vi "SENS_SWE_GEN.vi"(0 "VISA IN":refnum<visa-resource-name>, 1 "Source Frq. Mode":string(combo)="STEPped", 5 "error in":errorcluster, 7 "Channel":i32=1) -> (14 "VISA Out":refnum<visa-resource-name>, 19 "error out":errorcluster)   [LabVIEW 2018, in "PNA-X.lvlib"]
doc: "SENSe<cnum>:SWEep:GENeration <char> \n(Read-Write) Sets sweep as Stepped or Analog. \nParameters \n<cnum> Any existing channel number. If unspecified, value is set to 1 \n<char> Choose from: \nSTEPped - source frequency is CONSTANT during measurement of eah displayed \npoint. More accurate than ANALog. Dwell time can be set in this mode. \nANALog - source frequency is continuously RAMPING during measurement of each \ndisplayed point. Faster than STEPped. Sweep time (not dwell time) can be set in this \nmode. \nExamples SENS:SWE:GEN STEP \nsense2:sweep:generation analog \nQuery Syntax SENSe<cnum>:SWEep:GENeration? \nReturn Type Character"
uses:
  PNA-X.lvlib
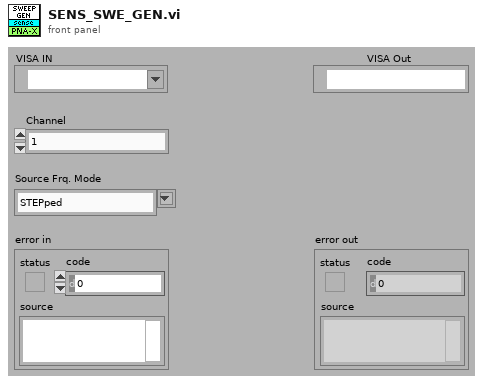
[diagram p1: front panel]
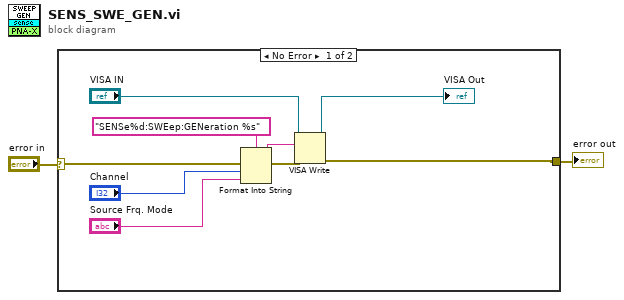
[diagram p0: block diagram]
diagram:
  n1 = case shown="No Error" "error in" {
    selector: "error in" -> [w11 w12]
    tunnel: [w6 w12] -> w1
    frame No Error {
      n2 = Format Into String(format string="SENSe%d:SWEep:GENeration %s" ("Cmdline"), error in=w11, "Channel", "Source Frq. Mode") -> (resulting string=w9:string, error out=w10:errorcluster)  [unwired: 1 in]
      n3 = VISA Write(VISA resource name="VISA IN", write buffer=w9, error in (no error)=w10) -> (VISA resource name out=→"VISA Out":refnum<visa-resource-name>, error out=w6:errorcluster)  [unwired: 1 out]
    }
    frame Error {
    }
  }
  "error out" <- w1
